vi "Motors Position Redefine.vi"(5 "Axis Multiplier":u32, 7 "Axis":u32, 8 "error in":errorcluster, 9 "VISA in":refnum<visa-resource-name>, 11 "Position (mm or deg)":dbl) -> (0 "error out":errorcluster, 1 "VISA out":refnum<visa-resource-name>)   [LabVIEW 2018]
panel:
  out "AP":string
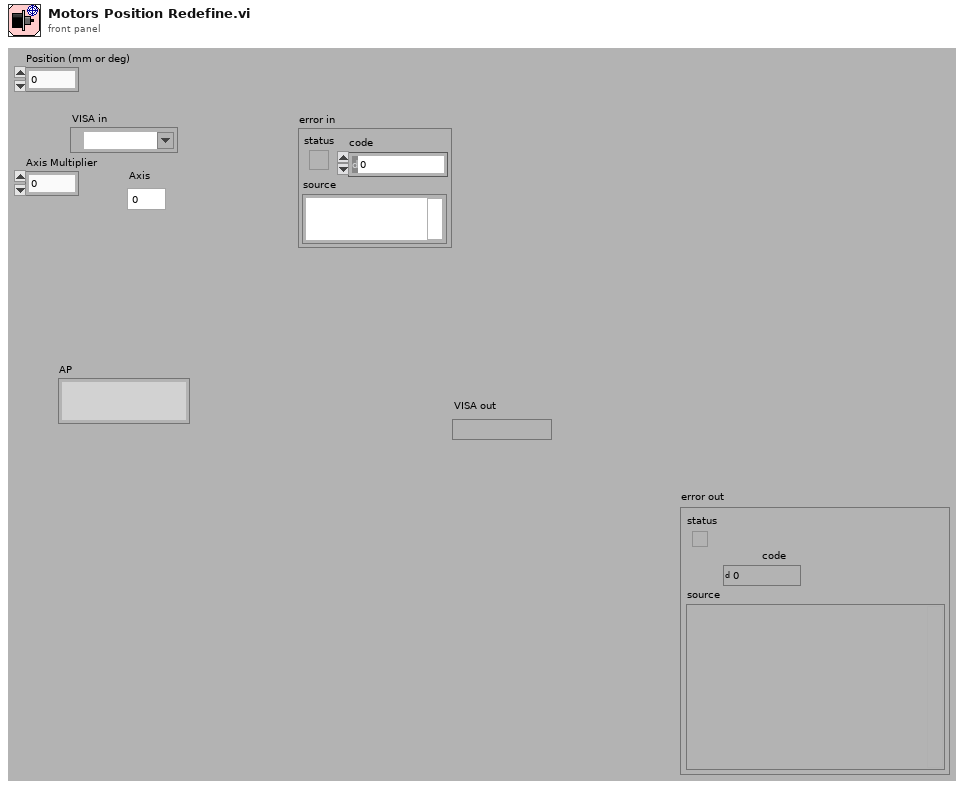
[diagram p1: front panel]
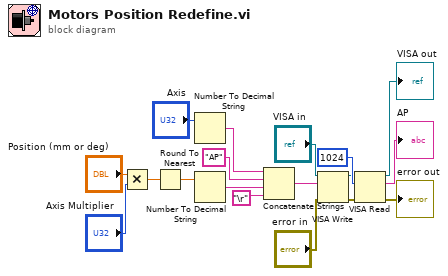
[diagram p0: block diagram]
diagram:
  n1 = Multiply(x="Position (mm or deg)", y="Axis Multiplier") -> (x*y=w9:dbl)
  n2 = Round To Nearest(number=w9) -> (nearest integer value=w10:dbl)
  n3 = Number To Decimal String(number="Axis") -> (decimal integer string=w4:string)  [unwired: 1 in]
  n4 = Number To Decimal String(number=w10) -> (decimal integer string=w3:string)  [unwired: 1 in]
  n5 = Concatenate Strings(w4, "AP" ("Initial command 3"), w3, "\r") -> (w15:string)
  n6 = VISA Write(VISA resource name="VISA in", write buffer=w15, error in (no error)="error in") -> (VISA resource name out=w13:refnum<visa-resource-name>, error out=w14:errorcluster)  [unwired: 1 out]
  n7 = VISA Read(VISA resource name=w13, byte count=u32 1024, error in (no error)=w14) -> (VISA resource name out=→"VISA out":refnum<visa-resource-name>, read buffer=→"AP":string, error out=→"error out":errorcluster)  [unwired: 1 out]
